vi "Angle Cluster from Points.vi"() -> ()   [LabVIEW 2017]
panel:
  out "appended array":T1(array[cluster])
  in  "Points":cluster{"X":dbl, "Y":dbl}[](array[cluster])
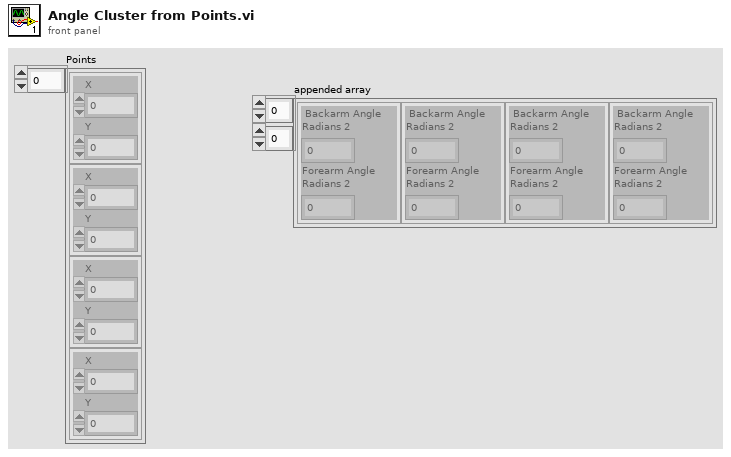
[diagram p1: front panel]
types:
  T1 = cluster{" Backarm Angle\nRadians 2":dbl, "Forearm Angle\nRadians 2":dbl}[][]
  T2 = cluster{" Backarm Angle\nRadians 2":dbl, "Forearm Angle\nRadians 2":dbl}
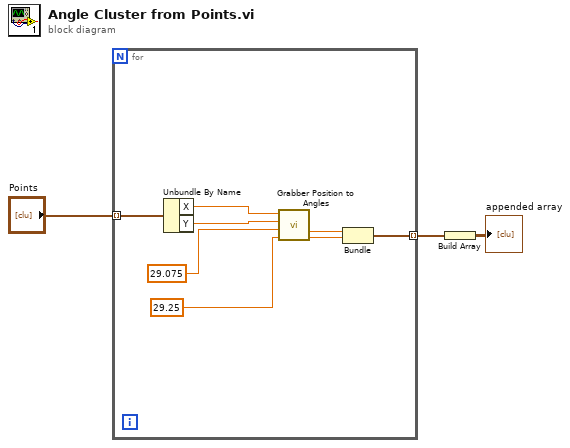
[diagram p0: block diagram]
diagram:
  n1 = for {
    tunnel: "Points" -> [w11] mode=indexing
    tunnel: [w4] -> w2 mode=indexing
    n2 = Unbundle By Name(w11) -> ("X"=w10:dbl, "Y"=w9:dbl)
    n3 = call "Grabber Position to Angles.vi"("Forearm Length"=29.25, "Backarm Length"=29.075, "Y Initial"=w9, "X Initial"=w10) -> ("Forearm Angle\nRadians 2"=w5:dbl, "Backarm Angle\nRadians 2"=w6:dbl)  [unwired: 4 in, 2 out]
    n4 = Bundle("Backarm Angle\nRadians 2"=w6, "Forearm Angle\nRadians 2"=w5) -> (w4:T2)  [unwired: 1 in]
  }
  n5 = Build Array(w2) -> (→"appended array":T1)
